vi "Initialize Daemon.vi"(8 "error in":errorcluster, 9 "Device Data Model":refnum<class "Device Data Model.lvclass">, 11 "network slave in":refnum<class "WebSocket Server.lvclass">) -> (0 "error out":errorcluster, 3 "network slave out":refnum<class "WebSocket Server.lvclass">)   [LabVIEW 2021, in "WebSockets.lvlib" / "WebSocket Server.lvclass"]
doc: "This provides an interface for the slave to launch a protocol daemon."
uses:
  WebSocket Server.lvclass
  Modbus_v121c/Data Model/Device Data Model.lvclass
  daemon status cluster.ctl
  daemon status.ctl
  WebSocket Server.lvclass/WebSocket Server.ctl
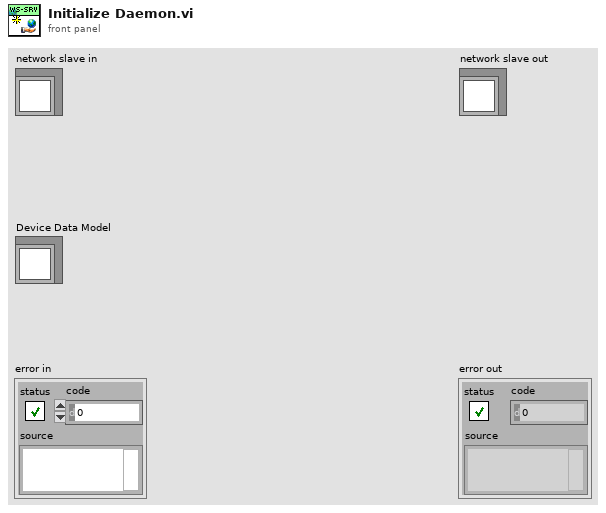
[diagram p1: front panel]
types:
  T1 = typedef "WebSockets.lvlib/WebSocket Server.lvclass/daemon status cluster.ctl" = cluster{"error":errorcluster, "status":T2}
  T2 = typedef "WebSockets.lvlib/WebSocket Server.lvclass/daemon status.ctl" = enum16{"Not Started", "Running", "Error", "Stopped"}
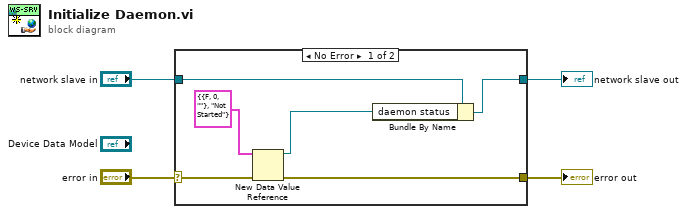
[diagram p0: block diagram]
diagram:
  n1 = case shown="No Error" "error in" {
    selector: "error in" -> [w8 w12]
    tunnel: "network slave in" -> [w10 w11]
    tunnel: [w9 w11] -> w2
    tunnel: [w6 w12] -> w1
    frame No Error {
      n2 = New Data Value Reference(data value=T1 {"error"={"status"=FALSE, "code"=0, "source"=""}, "status"=enum."Not Started"} ("Status"), error in=w8) -> (data value reference=w5:refnum<data-value>, error out=w6:errorcluster)
      n3 = Bundle By Name(cluster=w10, "daemon status"=w5) -> (w9:refnum<class "WebSocket Server.lvclass">)
    }
    frame Error {
    }
  }
  "error out" <- w1
  "network slave out" <- w2
